vi "Get DefaultValue+.vi"(8 "Error In":errorcluster, 11 "reference in":refnum<class "OD Entry.lvclass">) -> (0 "Error Out":errorcluster, 1 "Defined?":bool, 2 "DefaultValue":string, 3 "reference out":refnum<class "OD Entry.lvclass">)   [LabVIEW 2019, in "Electronic Datasheet.lvlib" / "OD Entry.lvclass"]
uses:
  OD Entry.lvclass
  Object Type/Object Type Base.lvclass
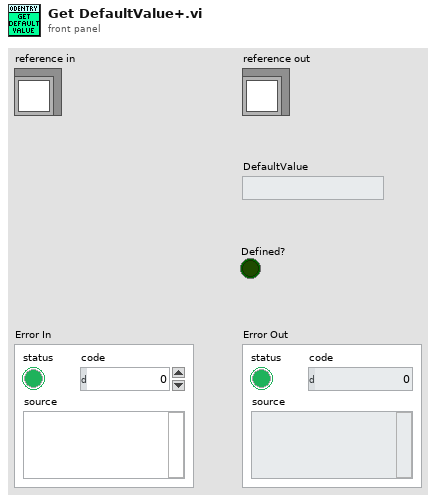
[diagram p1: front panel]
types:
  T1 = typedef "Electronic Datasheet.lvlib/OD Entry.lvclass/ObjectAttributes.ctl" = cluster{"Index":u16, "ObjectType":refnum<class "Object Type Base.lvclass">, "Denotation":string, "Count":u8, "ObjExtend":u8, "Label":string, "Description":string, "PDO Mapping Type":T2, "Sub-Entries":map{u8, refnum<class "OD Sub-Entry.lvclass">}}
  T2 = typedef "Electronic Datasheet.lvlib/PDO Mapping Type.ctl" = enum16{"no", "optional", "RPDO", "TPDO", "UNKNOWN"}
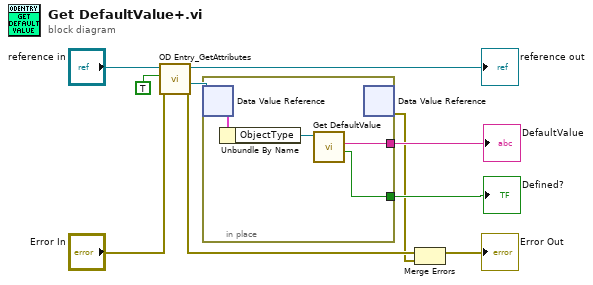
[diagram p0: block diagram]
diagram:
  n1 = call "OD Entry_GetAttributes.vi"("Error In"="Error In", "OnlyGetDvrReference(False)"=TRUE, "reference in"="reference in") -> ("Error Out"=w4:errorcluster, "DataRef"=w1:refnum<data-value>, "reference out"=→"reference out":refnum<class "OD Entry.lvclass">)  [unwired: 5 in, 1 out]
  n2 = in-place {
    in-place-border: [w12] -> w6
    in-place-border: [w11] -> w5
    n3 = in-place-dvr #1(w1) -> (w13:T1)  [unwired: 1 out]
    n4 = Unbundle By Name(w13) -> ("ObjectType"=w14:refnum<class "Object Type Base.lvclass">)
    n5 = call-dynamic "Get DefaultValue.vi"("Object Type in"=w14) -> ("Defined?"=w11:bool, "DefaultValue"=w12:string)  [unwired: 8 in, 1 out]
    n6 = in-place-dvr #1() -> (w3:errorcluster)  [unwired: 1 in, 1 out]
  }
  "DefaultValue" <- w6
  "Defined?" <- w5
  n7 = Merge Errors(w4, w3) -> (→"Error Out":errorcluster)
